vi "IMAQdx ROI.vi"() -> ()   [LabVIEW 2020]
uses:
  <vilib>/userDefined/High Color/IMAQdx.ctl
  <vilib>/vision/driver/NI_Vision_Acquisition_Software.lvlib
panel:
  out "Actual ROI":T1
  in  "Desired ROI":T1={"OffsetX"=0, "OffsetY"=0, "Width"=2560, "Height"=2048}
  in  "Capture Mode":enum16{"Continuously", "One Frame"}(ring)
  in  "Write in Continuous Mode":bool
  out "error out":errorcluster
  in  "error in":errorcluster
  in  "Stop Continuous Snap":bool
  in  "Session In":T2
  out "Image":T3(plugin-control)
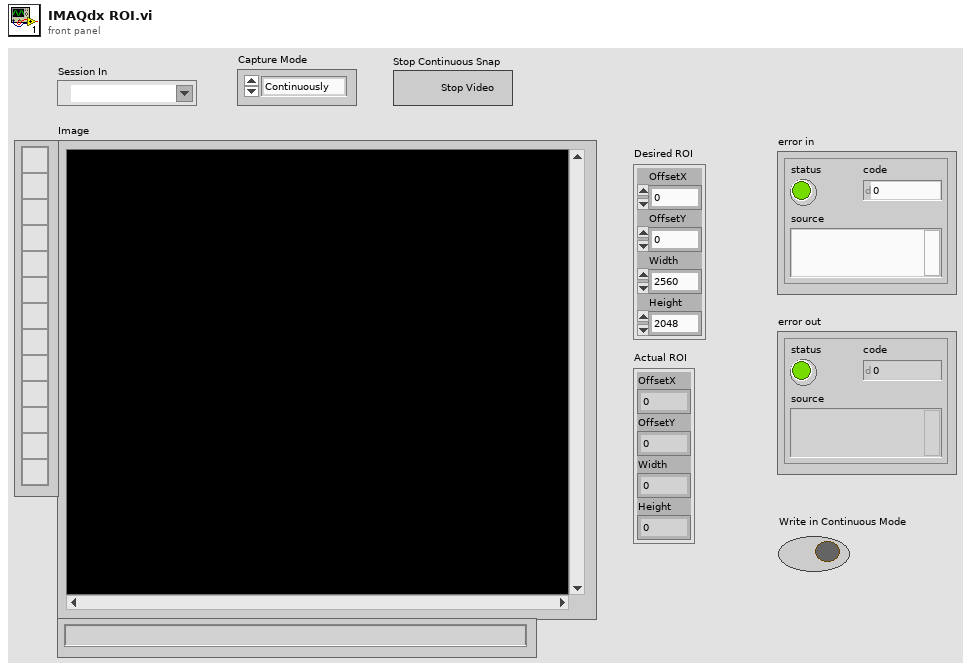
[diagram p1: front panel]
types:
  T1 = cluster{"OffsetX":i64, "OffsetY":i64, "Width":i64, "Height":i64}
  T2 = typedef "IMAQdx.ctl" = refnum<k21>
  T3 = typedef "IMAQ Image.ctl" = refnum<image>
  T4 = enum8{"Enabled", "Disabled", "Disabled and Grayed Out"}
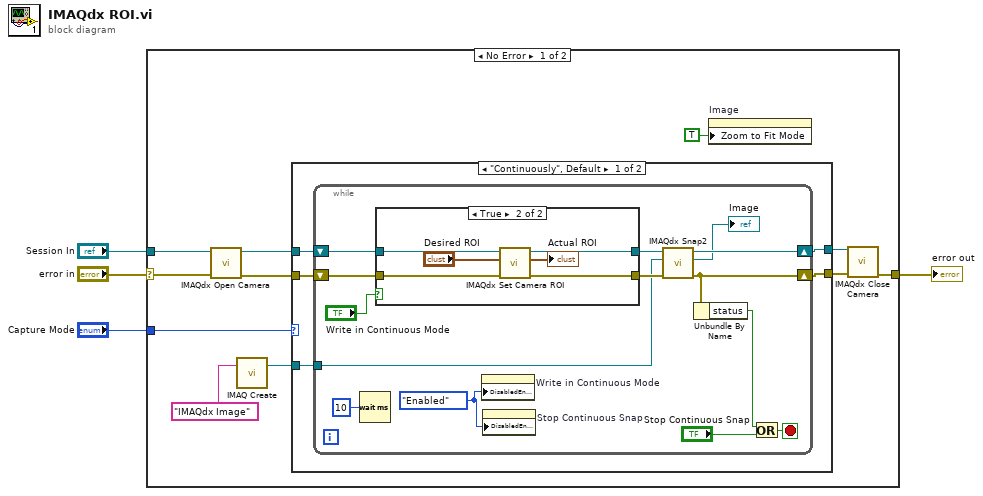
[diagram p0: block diagram]
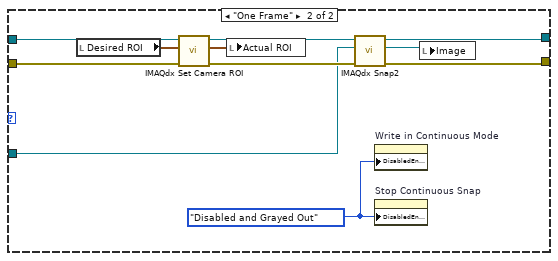
[diagram p3: hidden frame]
diagram:
  n1 = case shown="No Error" "error in" {
    selector: "error in" -> [w13 w54]
    tunnel: "Session In" -> [w14 _]
    tunnel: [w8 w54] -> w2
    tunnel: "Capture Mode" -> [w5 _]
    frame No Error {
      n2 = call <vilib>:"IMAQdx Open Camera.vi"("error in"=w13, "Session In"=w14) -> ("error out"=w12:errorcluster, "Session Out"=w7:T2)  [unwired: 8 in]
      n3 = call "IMAQ Create"("Image Name"="IMAQdx Image") -> ("New Image"=w11:T3)  [unwired: 4 in, 1 out]
      n4 = case shown="\"Continuously\", Default" w5 {
        tunnel: w12 -> [w20 w45]
        tunnel: w11 -> [w19 w50]
        tunnel: [w18 w52] -> w10
        tunnel: [w17 w51] -> w9
        tunnel: w7 -> [w16 w47]
        frame "Continuously", Default {
          n5 = while {
            shift-right: [w31] -> w18
            shift-left: w16 -> [w22]
            shift-right: [w27] -> w17
            shift-left: w20 -> [w21]
            tunnel: w19 -> [w28]
            stop <- w26 stop-if-true
            w23 = T4."Enabled" ("Disabled")
            n6 = Wait (ms)(milliseconds to wait=u32 10) -> ()  [unwired: 1 out]
            n7 = case shown="True" "Write in Continuous Mode" {
              tunnel: [w35 w41] -> w32
              tunnel: [w36 w40] -> w30
              tunnel: w22 -> [w35 w42]
              tunnel: w21 -> [w36 w39]
              frame False {
              }
              frame True {
                n8 = call "IMAQdx Set Camera ROI.vi"("error in (no error)"=w39, "Desired ROI"="Desired ROI", "Session in"=w42) -> ("error out"=w40:errorcluster, "Actual ROI"=→"Actual ROI":T1, "Session out"=w41:T2)  [unwired: 6 in]
              }
            }
            n9 = property on="Write in Continuous Mode" class="Bool (strict)"("DisabledEnum"=w23) -> ()  [unwired: 2 in, 2 out]
            n10 = property on="Stop Continuous Snap" class="Bool"("DisabledEnum"=w23) -> ()  [unwired: 2 in, 2 out]
            n11 = call <vilib>:"IMAQdx Snap2.vi"("error in"=w30, "Image In"=w28, "Session In"=w32) -> ("error out"=w27:errorcluster, "Image Out"=→"Image":T3, "Session Out"=w31:T2)  [unwired: 6 in]
            n12 = Unbundle By Name(w27) -> ("status"=w24:bool)
            n13 = Or(x=w24, y="Stop Continuous Snap") -> (x .or. y?=w26:bool)
          }
        }
        frame "One Frame" {
          w48 = T4."Disabled and Grayed Out" ("Disabled")
          n14 = local read "Desired ROI"() -> (w44:T1)
          n15 = call "IMAQdx Set Camera ROI.vi"("error in (no error)"=w45, "Desired ROI"=w44, "Session in"=w47) -> ("error out"=w53:errorcluster, "Actual ROI"=w43:T1, "Session out"=w46:T2)  [unwired: 6 in]
          n16 = local write "Actual ROI"(w43) -> ()
          n17 = call <vilib>:"IMAQdx Snap2.vi"("error in"=w53, "Image In"=w50, "Session In"=w46) -> ("error out"=w51:errorcluster, "Image Out"=w49:T3, "Session Out"=w52:T2)  [unwired: 6 in]
          n18 = property on="Write in Continuous Mode" class="Bool (strict)"("DisabledEnum"=w48) -> ()  [unwired: 2 in, 2 out]
          n19 = property on="Stop Continuous Snap" class="Bool"("DisabledEnum"=w48) -> ()  [unwired: 2 in, 2 out]
          n20 = local write "Image"(w49) -> ()
        }
      }
      n21 = property on="Image" class="ImageControl"("Zoom to Fit Mode"=TRUE) -> ()  [unwired: 2 in, 2 out]
      n22 = call <vilib>:"IMAQdx Close Camera.vi"("error in"=w9, "Session In"=w10) -> ("error out"=w8:errorcluster)  [unwired: 9 in]
    }
    frame Error {
    }
  }
  "error out" <- w2
